vi "DestroyTask.vi"(8 "error in (no error)":errorcluster, 11 "DAQ_Module in":refnum<class "DAQ_Module.lvclass">) -> (0 "error out":errorcluster, 3 "DAQ_Module out":refnum<class "DAQ_Module.lvclass">)   [LabVIEW 2025, in "DAQ_Module.lvlib" / "DAQ_Module.lvclass"]
uses:
  DAQ_Module.lvclass
  DAQ_Module.lvclass/DAQ_Module.ctl
  <vilib>/ActorFramework/Message Enqueuer/Message Enqueuer.lvclass/Message Enqueuer.ctl
  <vilib>/ActorFramework/Message Enqueuer/Enqueue.vi
  <vilib>/ActorFramework/Stop Msg/Stop Msg.lvclass
  <vilib>/ActorFramework/Message Priority Queue/Priority Enqueue.vi
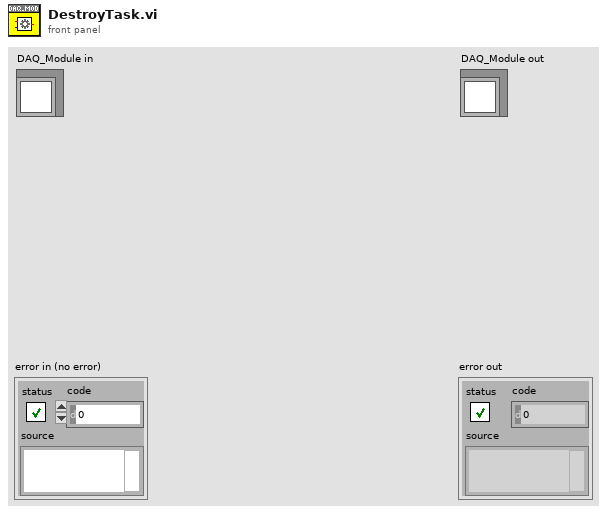
[diagram p1: front panel]
types:
  T1 = map{string, refnum<class "Message Enqueuer.lvclass">}
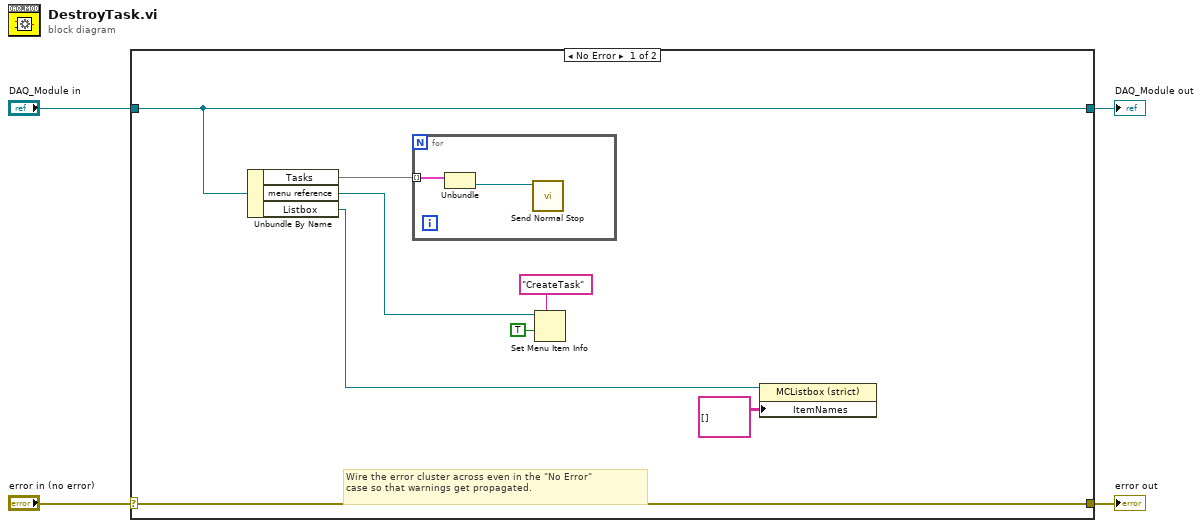
[diagram p0: block diagram]
diagram:
  n1 = case shown="No Error" "error in (no error)" {
    selector: "error in (no error)" -> [w12 w16]
    tunnel: [w12 w16] -> w3
    tunnel: [w11 w15] -> w1
    tunnel: "DAQ_Module in" -> [w11 w15]
    frame No Error {
      # "Wire the error cluster across even in the \"No Error\"\ncase so that warnings get propagated."
      n2 = Unbundle By Name(w11) -> ("Tasks"=w10:T1, "menu reference"=w7:refnum<k9>, "Listbox"=w6:refnum<vi>)
      n3 = for {
        tunnel: w10 -> [w14] mode=indexing
        n4 = Unbundle(w14) -> ("Nested Actor's Enqueuer"=w13:refnum<class "Message Enqueuer.lvclass">)  [unwired: 1 out]
        n5 = call <vilib>:"Send Normal Stop.vi"("Message Enqueuer"=w13) -> ()  [unwired: 10 in, 1 out]
      }
      n6 = Set Menu Item Info(7:"CreateTask" ("item tag"), 9:TRUE ("enabled"), 11:w7) -> ()  [unwired: 4 in, 2 out]
      n7 = property class="MCListbox (strict)"(reference=w6, "ItemNames"=string[][] [] ("Item Names")) -> ()  [unwired: 1 in, 2 out]
    }
    frame Error {
    }
  }
  "error out" <- w3
  "DAQ_Module out" <- w1
